vi "pullNodeFromOpen.vi"(8 "error in (no error)":errorcluster, 11 "Graph in":refnum<class "Graph.lvclass">) -> (0 "error out":errorcluster, 1 "empty":bool, 2 "RemovedNode":refnum<data-value>, 3 "Graph out":refnum<class "Graph.lvclass">)   [LabVIEW 2014, in "Graph.lvlib" / "Graph.lvclass"]
doc: "Pulls the first node off of OPEN. The first node is the node that is most likely to the be the goal node."
uses:
  <userlib>/AdvancedDataStructures/ClassBased/Graph/Graph.lvclass
  <userlib>/AdvancedDataStructures/ClassBased/LLNode/LLNode.lvclass
  <userlib>/AdvancedDataStructures/ClassBased/Graph/Graph.lvclass/Graph.ctl
  <userlib>/AdvancedDataStructures/ClassBased/LinkedList/position.ctl
  <userlib>/AdvancedDataStructures/ClassBased/LinkedList/LinkedList.lvclass
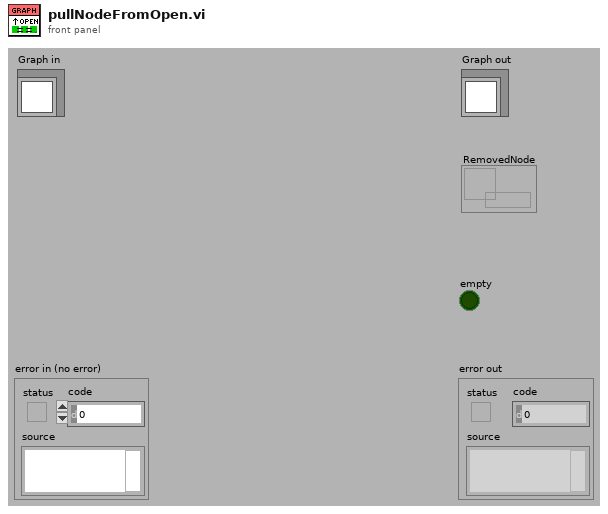
[diagram p1: front panel]
types:
  T1 = typedef "LinkedList.lvlib/LinkedList.lvclass/position.ctl" = enum16{"Front", "Back", "Search"}
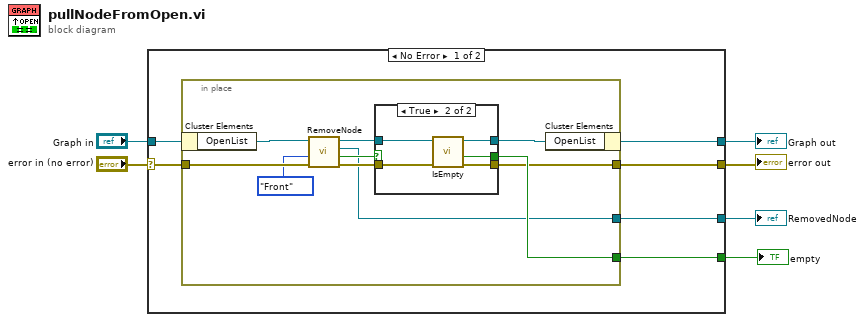
[diagram p0: block diagram]
diagram:
  n1 = case shown="No Error" "error in (no error)" {
    selector: "error in (no error)" -> [w11 w31]
    tunnel: [w8 w31] -> w3
    tunnel: [w9 w30] -> w4
    tunnel: "Graph in" -> [w12 w30]
    tunnel: [w10 _] -> w2
    tunnel: [w7 _] -> w1
    frame No Error {
      n2 = in-place {
        in-place-border: w11 -> [w21]
        in-place-border: [w16] -> w10
        in-place-border: [w15] -> w7
        in-place-border: [w13] -> w8
        n3 = in-place-cluster #1(w12) -> ("OpenList"=w22:refnum<class "BasicSortedList.lvclass">)
        n4 = call <userlib>:"RemoveNode.vi"("error in (no error)"=w21, "position"=position."Front", "LinkedList in"=w22) -> ("error out"=w17:errorcluster, "ignored"=w18:bool, "RemovedNode"=w15:refnum<data-value>, "LinkedList out"=w19:refnum<class "BasicSortedList.lvclass">)  [unwired: 5 in]
        n5 = case shown="True" w18 {
          tunnel: w19 -> [w24 w29]
          tunnel: w17 -> [w23 w28]
          tunnel: [_ w27] -> w16
          tunnel: [w24 w26] -> w14
          tunnel: [w23 w25] -> w13
          frame False {
          }
          frame True {
            n6 = call <userlib>:"IsEmpty.vi"("error in (no error)"=w28, "LinkedList in"=w29) -> ("error out"=w25:errorcluster, "empty"=w27:bool, "LinkedList out"=w26:refnum<class "BasicSortedList.lvclass">)  [unwired: 7 in]
          }
        }
        n7 = in-place-cluster #1("OpenList"=w14) -> (w9:refnum<class "Graph.lvclass">)
      }
    }
    frame Error {
    }
  }
  "error out" <- w3
  "Graph out" <- w4
  "empty" <- w2
  "RemovedNode" <- w1
